vi "SRV_XModem_Write File.vi"(8 "error in":errorcluster, 10 "file contents":string, 11 "connection ID in":refnum<k5>) -> (0 "error out":errorcluster, 1 "success?":bool, 2 "reply to upload":string="HTTP/1.1 200 OK\r\nContent-Type: image/jpeg\r\nCache-Control: no-cache\r\nPragma: no-cache\r\nConnection: Close\r\nContent-Length: 13047\r", 3 "connection ID":refnum<k5>, 6 "Replies":string[](array[string]))   [LabVIEW 2014]
doc: "Modified for Benilde St. Margaret's School - Tim Jump\nBy Doug Schmertman, Mike Schultz - Logic PD\nCopyright 2012"
uses:
  SRV_Package Methods.ctl
panel:
  out "reply":string
  out "Status":u8(slide) scale=0.0..100.0
  out "retries":u32[](graph)
  in  "Max Retries":i16=10
  out "interation":i32
  in  "XMODEM instructions":string="Perception presents:\n\n------------ Understanding The X-Modem File Transfer Protocol ---------------\n\n\n\n\t\t\t      by Em Decay\n\n\n\nThis has to be one of the most internationally accepted protocols for upload-\n\n ing and downloading binary and text files.  It is fairly straight-forward as\n\n to how it is set up and there are some error checking capablities.\n\n\n\n\n\n--- Before you begin ---\n\n\n\nThings you need to know beforehand...\n\n\n\nThe following terms are simply ascii codes:\n\n    SOH = chr(1)  = CTRL-A =\n\n    EOT = chr(4)  = CTRL-D = End of Transmission\n\n    ACK = chr(6)  = CTRL-F = Positive Acknowledgement\n\n    NAK = chr(21) = CTRL-U = Negative Acknowledgement\n\n    CAN = chr(24) = CTRL-X = Cancel\n\n\n\nIn order to send the file, you must first divide it into 128 byte sections\n\n (packets).  Bytes 0-127 of the file make up the first packet, bytes 128-255\n\n make up the second packet, etc.\n\n\n\nThe packet number sent is simply the number of the packet.  If the packet\n\n number is greater than 255, then subtract 256 repeatly until the number is\n\n between 0 and 255.  For example, if you were sending packet 731, then you\n\n would send 731 - 256 - 256 = 219.\n\n\n\nThe 1's complement of a byte (to make life easy) is simply 255 minus the\n\n byte.  For example, if you had to take the 1's complement of 142, the answer\n\n would be 255 - 142 = 133.\n\n\n\nThe checksum is the value of all the bytes in the packet added together.  For\n\n example, if the first five bytes were 45, 12, 64, 236, 173 and the other 123\n\n bytes were zeroes, the checksum would be 45+12+64+236+173+0+0+...+0 = 530.\n\n However, to make each block one byte smaller, they repeatly subtract 256\n\n from the checksum until it is between 0 and 255.  In this case, the checksum\n\n would be 530 - 256 - 256 = 18.\n\n\n\nThe first byte the downloader sends is referred to as the NCGbyte.\n\n\n\nProvided that you aren't lost already, here is what happens next.  The steps\n\n below describe who sends what when :)\n\n\n\n\n\n--- The Actual Transfer ---\n\n\n\nThe uploader waits until the downloader sends a NAK byte.  The NAK byte\n\n is the signal that the downloader is ready to start.  This byte is referred\n\n to as the NCGbyte.  If the downloader takes too long or an error occurs then \n\n the uploader will stop waiting or \"Time Out\".  If this happens, then the \n\n file transfer must restart.\n\n\n\nWith each packet sent...\n\n\n\n    The uploader sends:\n\n\n\n    1. an SOH byte                             {1 byte}\n\n    2. the packet number                       {1 byte}\n\n    3. the 1's complement of the packet number {1 byte}\n\n    4. the packet                            {128 bytes}\n\n    5. the checksum                            {1 byte}\n\n    The above five things are called the block.\n\n\n\n    The downloader:\n\n\n\n    1. ensures that the packet number sent matches the actual packet number\n\n\t that it is (If the third block send has a '4' as the second byte,\n\n\t something is wrong --> CANCEL TRANSFER (send CAN byte))\n\n    2. adds the packet number and the 1's complement of it together to make\n\n\t sure that they add up to 255.  if they don't --> CANCEL TRANSFER\n\n    3. adds up all the bytes in the packet together --> THE SUM\n\n    4. compares the last two significant digits of THE SUM with the checksum\n\n    5. if everything looks ok (sum=checksum), then the downloader appends the\n\n\t bytes in the packet to the file being created (sent).  The down-\n\n\t loader then sends an ACK byte which tells the uploader to send the\n\n\t next block.\n\n       if the sums do not match then the downloader sends an NAK byte which\n\n\t tells the uploader to send the same block it just sent over again.\n\n\n\nWhen the uploader sends an EOT byte instead of an SOH byte, the downloader\n\n sends a NAK byte.  If the uploader sends another EOT immediately after that,\n\n the downloader sends an ACK byte and the transfer is complete.\n\n\n\nAnother thing, the downloader can cancel the transfer at any time by sending\n\n a CAN byte.  The uploader can only cancel between blocks by sending a CAN\n\n byte.  It is recommended that you send anywhere between 2 and 8 consecutive\n\n CAN bytes when you wish to cancel as some programs will not let you abort if\n\n only 1 CAN byte is sent.\n\n\n\n\n\n--- Wrap Up ---\n\n\n\nHopefully, you were able to follow along. :)  If not, you can e-mail me at\n\n em_decay@norlink.net  and I will try to clarify it for you.  Have fun :)\n\n\n\nPerception:    Em Decay -- Mark Korhonen\n\n\t       Cmf ------- Chris Fillion\n\n\n\nWritten on Dec.28/95\n\n"
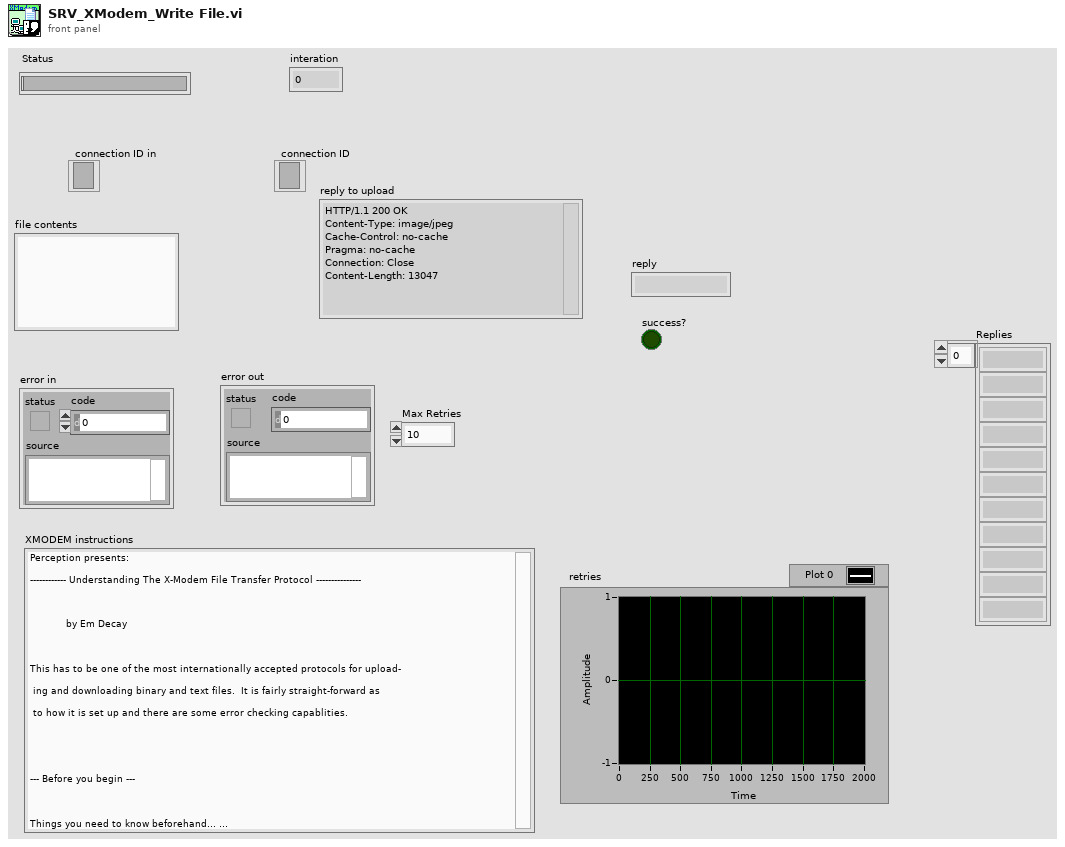
[diagram p1: front panel]
types:
  T1 = cluster{"bytes to read":i32, "msec pause":u32, "msec timeout":i32}
  T2 = typedef "SRV_Package Methods.ctl" = enum16{"General", "Standard", "CRLF", "Image", "HTML"}
  T3 = cluster{"SOH byte":u8, "Packet Number":u8, "Complement":u8, "Packet":u8[], "CRC":u8[], "FP":string}
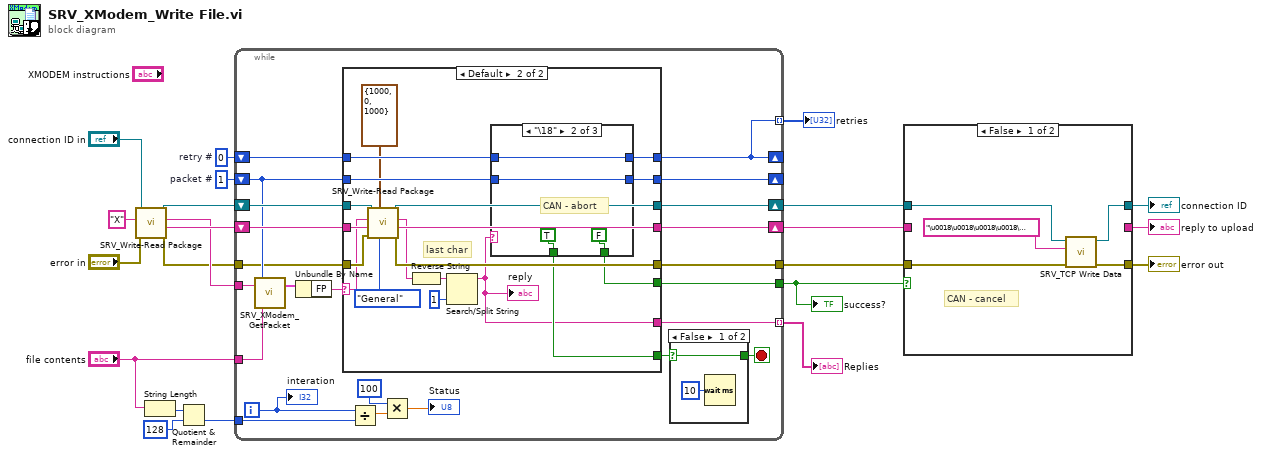
[diagram p0: block diagram]
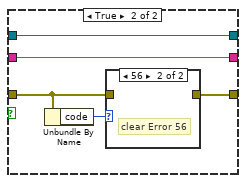
[diagram p2: hidden frame]
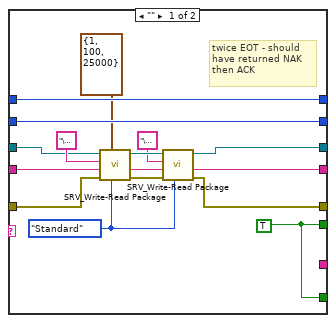
[diagram p5: hidden frame]
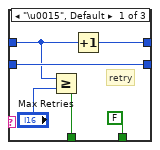
[diagram p6: hidden frame]
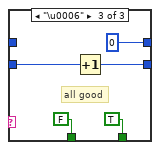
[diagram p7: hidden frame]
diagram:
  w16 = 1  # packet #
  w17 = u32 0  # retry #
  n1 = call "SRV_Write-Read Package.vi"("error in"="error in", "data in"="X", "connection ID in"="connection ID in") -> ("error out"=w11:errorcluster, "listing out"=w18:string, "data out"=w13:string, "connection ID"=w20:refnum<k5>)  [unwired: 5 in]
  n2 = String Length(string="file contents") -> (length=w7:i32)
  n3 = Quotient & Remainder(x=w7, y=128) -> (floor(x/y)=w5:i32)  [unwired: 1 out]
  n4 = while {
    shift-right: [w43] -> w15
    shift-left: w20 -> [w45]
    shift-right: [w42] -> w12
    shift-left: w18 -> [w44]
    shift-right: [w32] -> _
    shift-left: w17 -> [w38]
    shift-right: [w39] -> _
    shift-left: w16 -> [w40]
    tunnel: "file contents" -> [w34]
    tunnel: w11 -> [w37]
    tunnel: [w36] -> w9
    tunnel: [w35] -> w3
    tunnel: [w32] -> w14 mode=indexing
    tunnel: w13 -> [w31]
    tunnel: w5 -> [w30]
    tunnel: [w25] -> w1 mode=indexing
    i -> [w26]
    stop <- w23 stop-if-true
    n5 = call "SRV_XModem_GetPacket.vi"("text"=w34, "X reply"=w31, "packet #"=w40) -> ("Block"=w41:T3)  [unwired: 1 in]
    n6 = Unbundle By Name(w41) -> ("FP"=w33:string)
    n7 = case shown="Default" w33 {
      selector: w33 -> [_ w65]
      tunnel: w45 -> [w61 w83]
      tunnel: w44 -> [w58 w82]
      tunnel: [w59 w81] -> w43
      tunnel: [w56 w80] -> w42
      tunnel: [w64 w79] -> w32
      tunnel: w40 -> [w63 w78]
      tunnel: [w63 w77] -> w39
      tunnel: w38 -> [w64 w76]
      tunnel: w37 -> [w54 w75]
      tunnel: [w52 w74] -> w36
      tunnel: [w50 w73] -> w24
      tunnel: [w50 w72] -> w35
      tunnel: [_ w67] -> w25
      frame "" {
        w49 = SRV_Package_Methods."Standard" ("Method")
        w50 = TRUE
        # "twice EOT - should\nhave returned NAK \nthen ACK"
        n8 = call "SRV_Write-Read Package.vi"("Method"=w49, "parameters"=T1 {"bytes to read"=1, "msec pause"=100, "msec timeout"=25000}, "error in"=w54, "listing in"=w58, "data in"="\u0004", "connection ID in"=w61) -> ("error out"=w53:errorcluster, "listing out"=w57:string, "connection ID"=w60:refnum<k5>)  [unwired: 2 in, 1 out]
        n9 = call "SRV_Write-Read Package.vi"("Method"=w49, "error in"=w53, "listing in"=w57, "data in"="\u0004", "connection ID in"=w60) -> ("error out"=w52:errorcluster, "listing out"=w56:string, "connection ID"=w59:refnum<k5>)  [unwired: 3 in, 1 out]
      }
      frame Default {
        # "last char"
        n10 = call "SRV_Write-Read Package.vi"("Method"=SRV_Package_Methods."General", "parameters"=T1 {"bytes to read"=1000, "msec pause"=0, "msec timeout"=1000}, "error in"=w75, "listing in"=w82, "data in"=w65, "connection ID in"=w83) -> ("error out"=w74:errorcluster, "listing out"=w80:string, "data out"=w71:string, "connection ID"=w81:refnum<k5>)  [unwired: 2 in]
        n11 = Reverse String(1:w71) -> (0:w69:string)
        n12 = Search/Split String(string=w69, offset (0)=1) -> (substring before match=w67:string)  [unwired: 1 in, 2 out]
        "reply" <- w67
        n13 = case shown="\"\\18\"" w67 {
          tunnel: [w89 w93 u32 0 ("milliseconds to wait")] -> w79
          tunnel: w78 -> [w88 w92 w97]
          tunnel: [w88 w92 w96] -> w77
          tunnel: w76 -> [w86 w93 _]
          tunnel: [w84 TRUE FALSE] -> w73
          tunnel: [FALSE FALSE TRUE] -> w72
          frame "\u0015", Default {
            # "retry"
            n14 = Greater Or Equal?(x=w86, y="Max Retries") -> (x >= y?=w84:bool)
            n15 = Increment(x=w86) -> (x+1=w89:u32)
          }
          frame "\u0018" {
            # "CAN - abort"
          }
          frame "\u0006" {
            # "all good"
            n16 = Increment(x=w97) -> (x+1=w96:i32)
          }
        }
      }
    }
    n17 = Divide(x=w26, y=w30) -> (x/y=w29:dbl)
    n18 = Multiply(x=100 ("y"), y=w29) -> (x*y=→"Status":dbl)
    n19 = case shown="False" w24 {
      selector: w24 -> [w47 w48]
      tunnel: [w47 w48] -> w23
      frame False {
        n20 = Wait (ms)(milliseconds to wait=u32 10) -> ()  [unwired: 1 out]
      }
      frame True {
      }
    }
    "interation" <- w26
  }
  "success?" <- w3
  "retries" <- w14
  "Replies" <- w1
  n21 = case shown="False" w3 {
    tunnel: w15 -> [w103 w108]
    tunnel: w12 -> [_ w107]
    tunnel: w9 -> [w101 w105]
    tunnel: [w100 w104] -> w4
    tunnel: [w99 w108] -> w10
    tunnel: [_ w107] -> w2
    frame False {
      # "CAN - cancel"
      n22 = call "SRV_TCP Write Data.vi"("error in"=w101, "data in"="\u0018\u0018\u0018\u0018\u0018\u0018\u0018\u0018", "connection ID"=w103) -> ("error out"=w100:errorcluster, "connection ID out"=w99:refnum<k5>)  [unwired: 6 in, 1 out]
    }
    frame True {
      n23 = Unbundle By Name(w105) -> ("code"=w106:i32)
      n24 = case shown="56" w106 {
        tunnel: [w109 _] -> w104
        tunnel: w105 -> [w109 _]
        frame Default {
        }
        frame 56 {
          # "clear Error 56"
        }
      }
    }
  }
  "connection ID" <- w10
  "error out" <- w4
  "reply to upload" <- w2
